vi "ph acquire instructiion.vi"() -> ()   [LabVIEW 2013]
uses:
  <vilib>/httpClient/LabVIEWHTTPClient.lvlib
panel:
  out "body":string
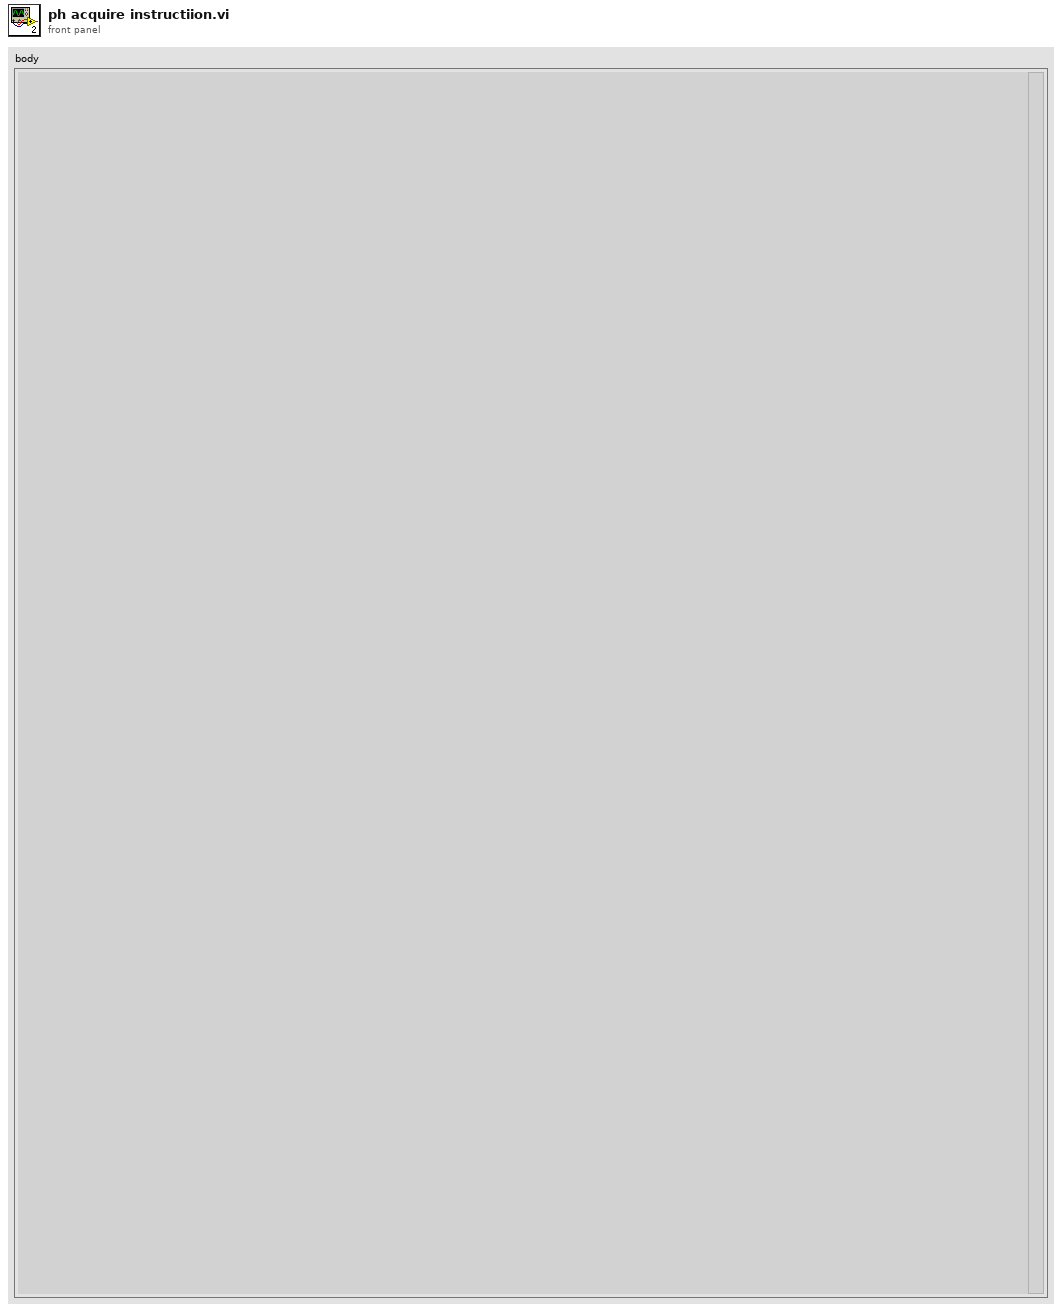
[diagram p1: front panel]
types:
  T1 = typedef "LabVIEWHTTPClient.lvlib/ClientHandle.ctl" = refnum<k1>
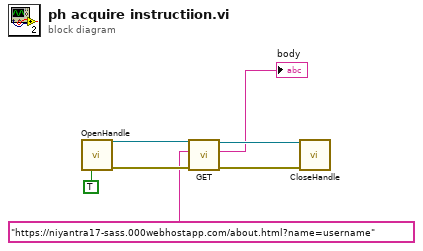
[diagram p0: block diagram]
diagram:
  n1 = call <vilib>:"OpenHandle.vi"("verify server(true)"=TRUE) -> ("client handle out"=w6:T1, "error out"=w5:errorcluster)  [unwired: 13 in]
  n2 = call <vilib>:"GET.vi"("client handle"=w6, "url"="https://niyantra17-sass.000webhostapp.com/about.html?name=username", "error in (no error)"=w5) -> ("client handle out"=w7:T1, "body"=→"body":string, "error out"=w4:errorcluster)  [unwired: 9 in, 1 out]
  n3 = call <vilib>:"CloseHandle.vi"("client handle"=w7, "error in (no error)"=w4) -> ()  [unwired: 13 in, 1 out]
